vi "GPS经纬度解析 (子VI).vi"(9 "数值输入":u16, 10 "数值 3":u16, 11 "数值 4":u16) -> (3 "数值输出":dbl format="%#.6g")   [LabVIEW 2016, in "环境动力监测库.lvlib" / "NMEA.lvlib"]
uses:
  NMEA.lvlib
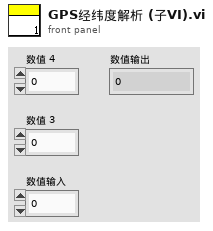
[diagram p1: front panel]
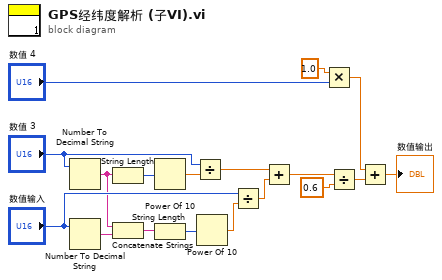
[diagram p0: block diagram]
diagram:
  n1 = Number To Decimal String(number="数值 3") -> (decimal integer string=w12:string)  [unwired: 1 in]
  n2 = Number To Decimal String(number="数值输入") -> (decimal integer string=w13:string)  [unwired: 1 in]
  n3 = String Length(string=w12) -> (length=w8:i32)
  n4 = Concatenate Strings(w12, w13) -> (w14:string)
  n5 = Power Of 10(x=w8) -> (10^x=w7:dbl)
  n6 = String Length(string=w14) -> (length=w15:i32)
  n7 = Divide(x="数值 3", y=w7) -> (x/y=w4:dbl)
  n8 = Power Of 10(x=w15) -> (10^x=w16:dbl)
  n9 = Divide(x="数值输入", y=w16) -> (x/y=w18:dbl)
  n10 = Add(x=w4, y=w18) -> (x+y=w6:dbl)
  n11 = Multiply(x=1.0, y="数值 4") -> (x*y=w2:dbl)
  n12 = Divide(x=w6, y=0.6) -> (x/y=w3:dbl)
  n13 = Add(x=w2, y=w3) -> (x+y=→"数值输出":dbl)
